vi "AutoLinker.vi"(8 "error in":errorcluster, 9 "format":string=".txt", 10 "filename":string="xy", 11 "Save Path":path) -> (0 "error out":errorcluster caption="error", 2 "DupFiles":bool, 3 "appended path":path)   [LabVIEW 2017]
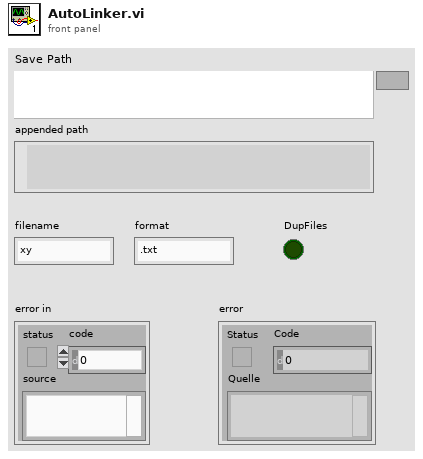
[diagram p1: front panel]
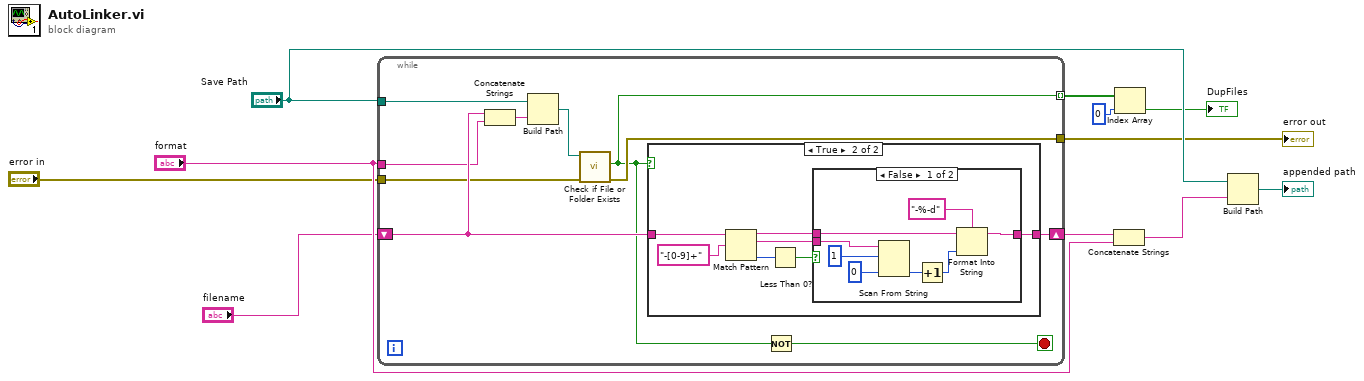
[diagram p0: block diagram]
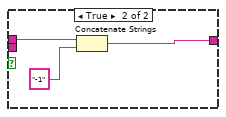
[diagram p3: hidden frame]
diagram:
  n1 = while {
    shift-right: [w19] -> w11
    shift-left: "filename" -> [w17]
    tunnel: "Save Path" -> [w16]
    tunnel: "format" -> [w15]
    tunnel: [w14] -> w5
    tunnel: "error in" -> [w13]
    tunnel: [w12] -> w3 mode=indexing
    stop <- w21 stop-if-true
    n2 = Concatenate Strings(w17, w15) -> (w18:string)
    n3 = Build Path(base path=w16, name or relative path=w18) -> (appended path=w20:path)
    n4 = call <vilib>:"Check if File or Folder Exists.vi"("error in (no error)"=w13, "path"=w20) -> ("error out"=w14:errorcluster, "file or folder exists?"=w12:bool)  [unwired: 7 in, 1 out]
    n5 = case shown="True" w12 {
      tunnel: w17 -> [w22 w29]
      tunnel: [w22 w24] -> w19
      frame False {
      }
      frame True {
        n6 = Match Pattern(string=w29, regular expression="-[0-9]+" ("正規表現")) -> (before substring=w25:string, match substring=w23:string, offset past match=w27:i32)  [unwired: 1 in, 1 out]
        n7 = Less Than 0?(x=w27) -> (x < 0?=w26:bool)
        n8 = case shown="False" w26 {
          tunnel: w25 -> [w32 w40]
          tunnel: [w30 w38] -> w24
          tunnel: w23 -> [w37 _]
          frame False {
            n9 = Scan From String(input string=w37, initial scan location=u32 1 ("初期スキャン位置"), default 1=u32 0 ("初期スキャン位置")) -> (output 1=w34:u32)  [unwired: 2 in, 3 out]
            n10 = Increment(x=w34) -> (x+1=w33:u32)
            n11 = Format Into String(format string="-%-d" ("形式文字列"), initial string=w32, w33) -> (resulting string=w30:string)  [unwired: 1 in, 1 out]
          }
          frame True {
            n12 = Concatenate Strings(w40, "-1") -> (w38:string)
          }
        }
      }
    }
    n13 = Not(x=w12) -> (.not. x?=w21:bool)
  }
  "error out" <- w5
  n14 = Concatenate Strings(w11, "format") -> (w10:string)
  n15 = Index Array(array=w3, index=0) -> (element=→"DupFiles":bool)
  n16 = Build Path(base path="Save Path", name or relative path=w10) -> (appended path=→"appended path":path)
